vi "Read IO_Data_Dir and IO_Data_Wr.vi"(8 "error in (no error)":errorcluster) -> (0 "error out":errorcluster, 2 "IO Data_Wr":u32[](array[numeric]), 3 "IO Data_Dir":u32)   [LabVIEW 2016]
uses:
  Host/Typedefs/IO Buffer Operation.ctl
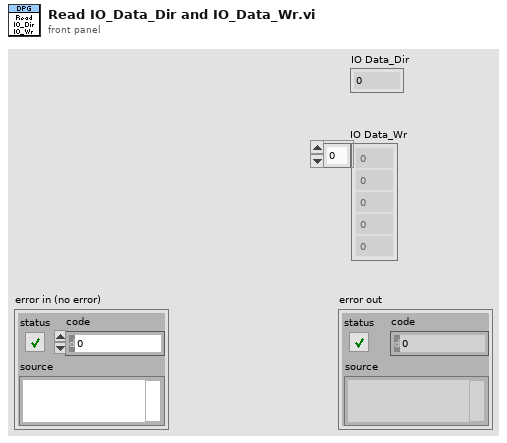
[diagram p1: front panel]
types:
  T1 = typedef "IO Buffer Operation.ctl" = enum16{"Initialize", "Write IO Data_Rd", "Read IO Data_Rd", "Write IO Data_Wr", "Read IO Data_Wr", "Write  IO Data_Dir", "Read  IO Data_Dir", "Write Host to Target FIFO", "Read Host to Target FIFO", "Write Target to Host FIFO", "Read Target to Host FIFO", "Write Monitor Enable?", "Read Monitor Enable?", "Close"}
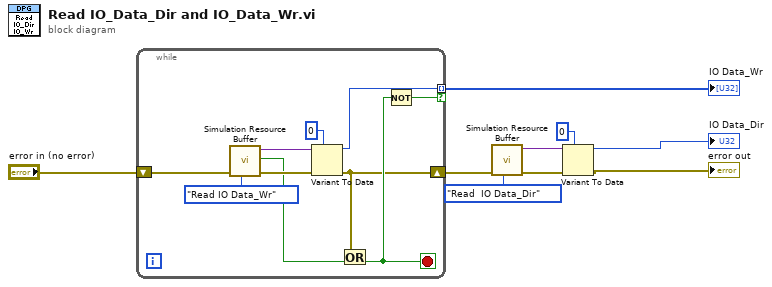
[diagram p0: block diagram]
diagram:
  n1 = while {
    tunnel: [w16] -> w9 mode=indexing if=w12
    shift-right: [w10] -> w6
    shift-left: "error in (no error)" -> [w15]
    stop <- w11 stop-if-true
    n2 = call "Simulation Resource Buffer.vi"("IO Buffer Operation"=IO_Buffer_Operation."Read IO Data_Wr", "error in (no error)"=w15) -> ("error out"=w18:errorcluster, "Timed Out?"=w13:bool, "Data out"=w17:variant)  [unwired: 7 in]
    n3 = Variant To Data(error in=w18, type=u32 0 ("Target to Host Data"), Variant=w17) -> (data=w16:u32, error out=w10:errorcluster)
    n4 = Or(x=w10, y=w13) -> (x .or. y?=w11:bool)
    n5 = Not(x=w11) -> (.not. x?=w12:bool)
  }
  "IO Data_Wr" <- w9
  n6 = call "Simulation Resource Buffer.vi"("IO Buffer Operation"=IO_Buffer_Operation."Read  IO Data_Dir", "error in (no error)"=w6) -> ("error out"=w4:errorcluster, "Data out"=w2:variant)  [unwired: 7 in, 1 out]
  n7 = Variant To Data(error in=w4, type=u32 0 ("Target to Host Data"), Variant=w2) -> (data=→"IO Data_Dir":u32, error out=→"error out":errorcluster)
